vi "Version_Destinations.vi"(8 "error in (no error)":errorcluster, 10 "include local destination":bool, 11 "Class in":refnum<class "AB_Build.lvclass">) -> (0 "error out":errorcluster, 3 "Class out":refnum<class "AB_Build.lvclass">)   [LabVIEW 2020, in "AB_Build.lvclass"]
uses:
  <vilib>/AppBuilder/AB_Classes/Build/AB_Build.lvclass
  <vilib>/AppBuilder/AB_Classes/Build/AB_Build.lvclass/AB_Build.ctl
  <vilib>/AppBuilder/RW_Project/AB_RW_Project_PropBag_Action.ctl
  <vilib>/AppBuilder/AB_Classes/Destination/AB_Destination.lvclass
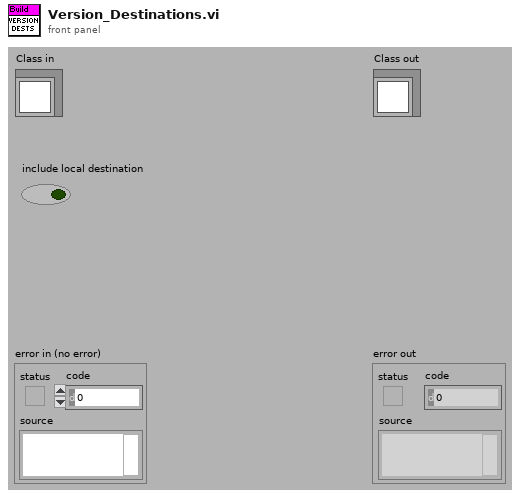
[diagram p1: front panel]
types:
  T1 = typedef "AB_RW_Project_PropBag_Action.ctl" = enum16{"read", "write", "clear", "readPrevious", "writePrevious", "clearPrevious"}
  T2 = typedef "ItemRef.ctl" = u64
  T3 = cluster{"major":u16, "minor":u16, "patch":u16, "build":u16}
  T4 = typedef "AB_RW_Project_Cache_Data.ctl" = cluster{"build preview data":T5, "project symbol checksum":string, "target symbol checksum":string, "My Computer checksum":string}
  T5 = typedef "build preview data.ctl" = cluster{"generated files":path[], "output directory":path, "buildVersion":cluster{"major":u16, "minor":u16, "patch":u16, "build":u16}}
  T6 = typedef "AB_Destination.ctl" = cluster{"destName":string, "path":path, "libraryName":string, "preserveHierarchy":bool, "eng_inBuild":bool, "eng_libraryReference":refnum<vi>, "eng_restictAddToNewLibrary":bool}
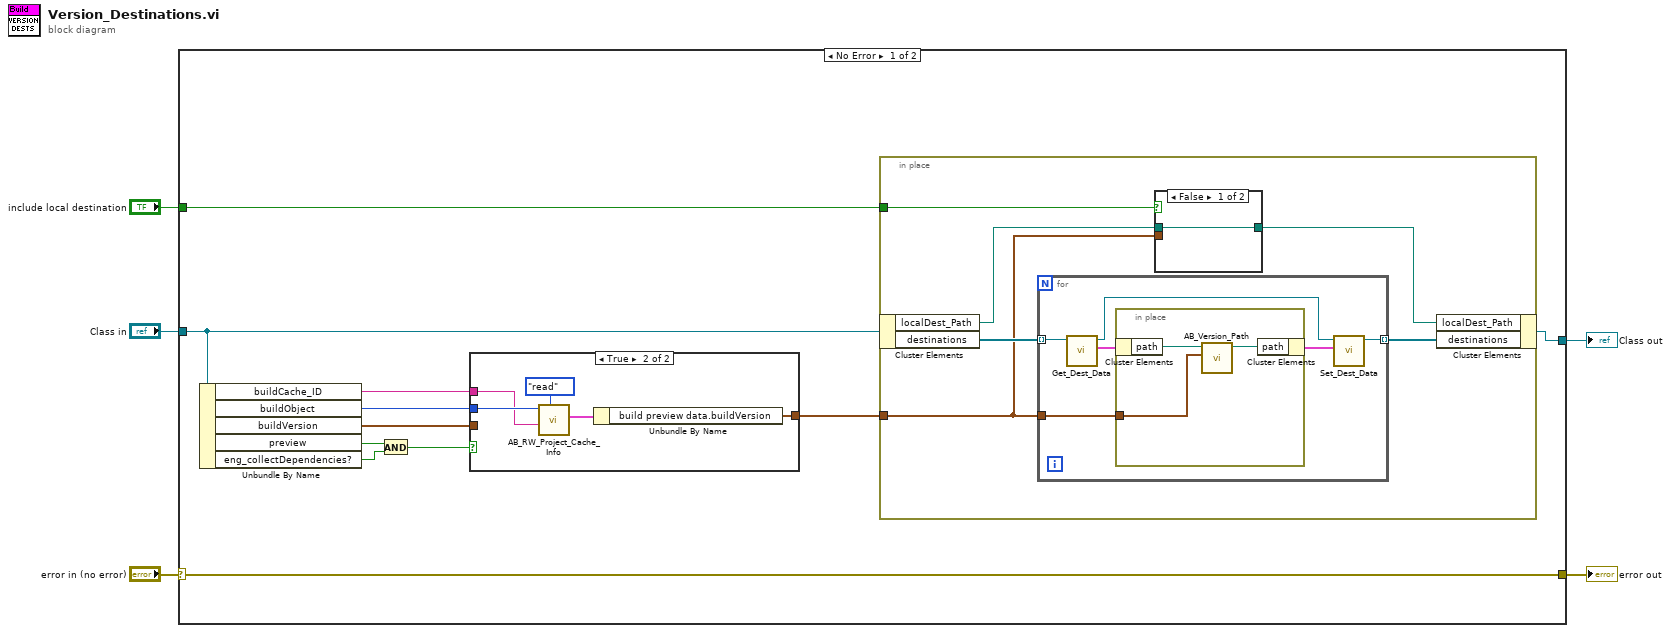
[diagram p0: block diagram]
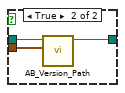
[diagram p3: hidden frame]
diagram:
  n1 = case "Case" shown="No Error" "error in (no error)" {
    selector: "error in (no error)" -> [w16 w43]
    tunnel: [w16 w43] -> w4
    tunnel: [w15 w42] -> w2
    tunnel: "Class in" -> [w14 w42]
    tunnel: "include local destination" -> [w6 _]
    frame No Error {
      n2 = Unbundle By Name(w14) -> ("buildCache_ID"=w7:string, "buildObject"=w13:T2, "buildVersion"=w8:T3, "preview"=w11:bool, "eng_collectDependencies?"=w10:bool)
      n3 = And(x=w11, y=w10) -> (x .and. y?=w9:bool)
      n4 = case shown="True" w9 {
        tunnel: w13 -> [_ w19]
        tunnel: [w17 w21] -> w12
        tunnel: w8 -> [w17 _]
        tunnel: w7 -> [_ w18]
        frame False {
        }
        frame True {
          n5 = call <vilib>:"AB_RW_Project_Cache_Info.vi"("action"=AB_RW_Project_PropBag_Action."read", "cache_ID"=w18, "Object In"=w19) -> ("info out"=w22:T4)  [unwired: 4 in, 4 out]
          n6 = Unbundle By Name(w22) -> ("build preview data.buildVersion"=w21:T3)
        }
      }
      n7 = in-place {
        in-place-border: w12 -> [w25]
        in-place-border: w6 -> [w23]
        n8 = in-place-cluster #1(w14) -> ("localDest_Path"=w26:path, "destinations"=w28:refnum<class "AB_Destination.lvclass">[])
        n9 = for {
          tunnel: w28 -> [w38] mode=indexing
          tunnel: w25 -> [w36]
          tunnel: [w33] -> w27 mode=indexing
          n10 = call <vilib>:"Get_Dest_Data.vi"("Class in"=w38) -> ("destName"=w37:T6, "Class out"=w35:refnum<class "AB_Destination.lvclass">)  [unwired: 8 in, 1 out]
          n11 = in-place {
            in-place-border: w36 -> [w39]
            n12 = in-place-cluster #2(w37) -> ("path"=w41:path)
            n13 = call <vilib>:"AB_Version_Path.vi"("buildVersion"=w39, "unversioned path"=w41) -> ("versioned path"=w40:path)  [unwired: 9 in]
            n14 = in-place-cluster #2("path"=w40) -> (w34:T6)
          }
          n15 = call <vilib>:"Set_Dest_Data.vi"("destName"=w34, "Class in"=w35) -> ("Class out"=w33:refnum<class "AB_Destination.lvclass">)  [unwired: 8 in, 1 out]
        }
        n16 = case shown="False" w23 {
          tunnel: w26 -> [w29 w32]
          tunnel: w25 -> [_ w31]
          tunnel: [w29 w30] -> w24
          frame False {
          }
          frame True {
            n17 = call <vilib>:"AB_Version_Path.vi"("buildVersion"=w31, "unversioned path"=w32) -> ("versioned path"=w30:path)  [unwired: 9 in]
          }
        }
        n18 = in-place-cluster #1("localDest_Path"=w24, "destinations"=w27) -> (w15:refnum<class "AB_Build.lvclass">)
      }
    }
    frame Error {
    }
  }
  "error out" <- w4
  "Class out" <- w2
